vi "0506_Identificador_QR.vi"() -> (27 "error out":errorcluster)   [LabVIEW 2017]
uses:
  <vilib>/userdefined/High Color/IMAQdx.ctl
  <vilib>/vision/Instrument.llb/QR Code Search Options.ctl
  <vilib>/vision/Instrument.llb/Demodulation Mode.ctl
  <vilib>/vision/Instrument.llb/Cell Sample Size.ctl
  <vilib>/vision/Instrument.llb/Cell Filter Mode.ctl
  <vilib>/vision/Instrument.llb/QR Code Description Options.ctl
  <vilib>/vision/Instrument.llb/Data Matrix Polarity.ctl
  <vilib>/vision/Instrument.llb/QR Code Model Type.ctl
  <vilib>/vision/driver/IMAQdx.llb/IMAQdx Acquisition Mode.ctl
  <vilib>/vision/driver/IMAQdx.llb/IMAQdx Buffer Number Mode.ctl
  <vilib>/vision/NI_Vision_Development_Module.lvlib
  <vilib>/vision/driver/NI_Vision_Acquisition_Software.lvlib
panel:
  out "Table Control":string[][](table)
  in  "Boolean":bool
  out "dt":dbl
  in  "QR Description Options":T1={"Matrix Size (cells)"=0, "Barcode Polarity"=-2, "Mirror Mode"=0, "QR Model"=3} {"Mirror Mode" items=["Auto-detect"=-2, "Normal"=0, "Mirrored"=1]; "Matrix Size (cells)" items=["Auto-detect"=0, "11x11 - Version 1 (Micro QR Only)"=11, "13x13 - Version 2 (Micro QR Only)"=13, "15x15 - Version 3 (Micro QR Only)"=15, "17x17 - Version 4 (Micro QR Only)"=17, "21x21 - Version 1"=21, "25x25 - Version 2"=25, "29x29 - Version 3"=29, "33x33 - Version 4"=33, "37x37 - Version 5"=37, "41x41 - Version 6"=41, "45x45 - Version 7"=45, "49x49 - Version 8"=49, "53x53 - Version 9"=53, "57x57 - Version 10"=57, "61x61 - Version 11"=61, "65x65 - Version 12"=65, "69x69 - Version 13"=69, "73x73 - Version 14"=73, "77x77 - Version 15"=77, "81x81 - Version 16"=81, "85x85 - Version 17"=85, "89x89 - Version 18"=89, "93x93 - Version 19"=93, "97x97 - Version 20"=97, "101x101 - Version 21"=101, "105x105 - Version 22"=105, "109x109 - Version 23"=109, "113x113 - Version 24"=113, "117x117 - Version 25"=117, "121x121 - Version 26"=121, "125x125 - Version 27"=125, "129x129 - Version 28"=129, "133x133 - Version 29"=133, "137x137 - Version 30"=137, "141x141 - Version 31"=141, "145x145 - Version 32"=145, "149x149 - Version 33"=149, "153x153 - Version 34"=153, "157x157 - Version 35"=157, "161x161 - Version 36"=161, "165x165 - Version 37"=165, "169x169 -  Version 38"=169, "173x173 - Version 39"=173, "177x177 - Version 40"=177]; "QR Model" items=["Auto-detect", "Micro", "Model 1", "Model 2"]; "Barcode Polarity" items=["Auto-detect"=-2, "Black on White"=0, "White on Black"=1]}
  in  "QR Search Options":T4={"Rotation Mode"=enum."Unlimited", "Skip Location?"=FALSE, "Edge Threshold"=30, "Demodulation Mode"=0, "Cell Sample Size"=-2, "Cell Filter Mode"=0, "Skew Degrees Allowed"=5} {"Cell Filter Mode" items=["Auto-detect"=-2, "Average"=0, "Median"=1, "Central Average"=2, "High Average"=3, "Low Average"=4, "Very High Average"=5, "Very Low Average"=6, "All Filters"=8]; "Cell Sample Size" items=["Auto-detect"=-2, "1x1"=1, "2x2"=2, "3x3"=3, "4x4"=4, "5x5"=5, "6x6"=6, "7x7"=7]; "Demodulation Mode" items=["Auto-detect"=-2, "Histogram"=0, "Local Contrast"=1, "Combination"=2, "All"=3]}
  in  "Threshold":cluster{"Lower value":sgl, "Upper value":sgl}={"Lower value"=0.0, "Upper value"=201.0219} {"Upper value" scale=0.0..255.0; "Lower value" scale=0.0..255.0}
  out "Image Out 2":T8(plugin-control)
  in  "Câmera":T9="cam1"
  in  "Stop Button":bool
  out "Image Out":T8(plugin-control)
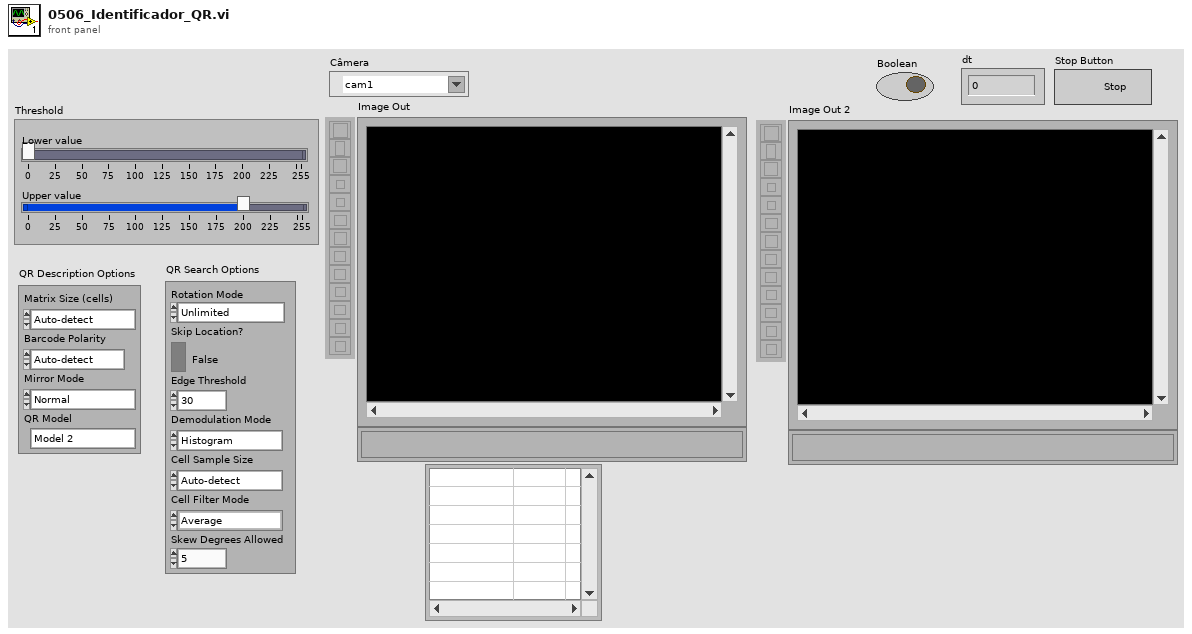
[diagram p1: front panel]
types:
  T1 = typedef "QR Code Description Options.ctl" = cluster{"Matrix Size (cells)":i32, "Barcode Polarity":T2, "Mirror Mode":i32, "QR Model":T3}
  T2 = typedef "Data Matrix Polarity.ctl" = i32
  T3 = typedef "QR Code Model Type.ctl" = i32
  T4 = typedef "QR Code Search Options.ctl" = cluster{"Rotation Mode":enum32{"Unlimited", "0 Degrees", "90 Degrees", "180 Degrees", "270 Degrees"}, "Skip Location?":bool, "Edge Threshold":u32, "Demodulation Mode":T5, "Cell Sample Size":T6, "Cell Filter Mode":T7, "Skew Degrees Allowed":u32}
  T5 = typedef "Demodulation Mode.ctl" = i32
  T6 = typedef "Cell Sample Size.ctl" = i32
  T7 = typedef "Cell Filter Mode.ctl" = i32
  T8 = typedef "IMAQ Image.ctl" = refnum<image>
  T9 = typedef "IMAQdx.ctl" = refnum<k21>
  T10 = typedef "Image Type" = u32
  T11 = typedef "NI_Vision_Acquisition_Software.lvlib/IMAQdx Acquisition Mode.ctl" = enum32{"One Shot", "Continuous"}
  T12 = typedef "NI_Vision_Acquisition_Software.lvlib/IMAQdx Buffer Number Mode.ctl" = enum32{"Next", "Last", "Buffer Number", "Every", "Last New"}
  T13 = cluster{"Global Rectangle":i32[], "Contours":cluster{"Contour Type":u32, "ROI Type":u32, "Points":i32[]}[]}
  T14 = typedef "QR Code Report.ctl" = cluster{"Found?":bool, "Data":string, "Bounding Box":cluster{"x":sgl, "y":sgl}[], "Errors Corrected":u32, "Dimensions (Rows/Cols)":u32, "Version":u32, "QR Model":T3, "Stream Mode":T15, "Barcode Polarity":T2, "Mirrored?":bool, "Append Stream Position":u32, "Size of Append Stream":u32, "First EAN-128 ID":i32, "First Alternate Language ID":i32, "Append Stream ID":u32, "Minimum Edge Strength":u32, "Demodulation Mode":T5, "Cell Sample Size":T6, "Cell Filter Mode":T7}
  T15 = typedef "QR Code Stream Mode Type.ctl" = i32
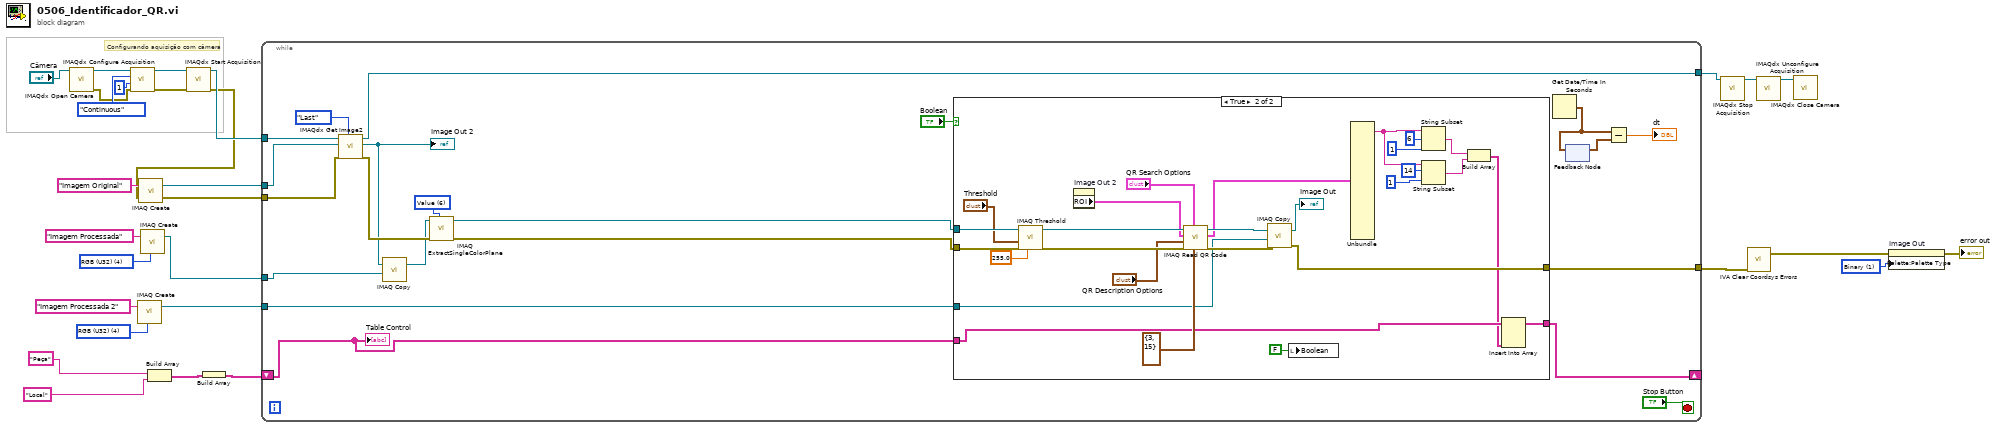
[diagram p0: block diagram]
diagram:
  w7 = T10 4 items=["Grayscale (U8)", "Grayscale (I16)", "Grayscale (SGL)", "Complex (CSG)", "RGB (U32)", "HSL (U32)", "RGB (U64)", "Grayscale (U16)"] ("Image Type")
  w14 = u32 1 items=["Grayscale", "Binary", "Gradient", "Rainbow", "Temperature", "User Defined", "Binary 16 Bit", "Gradient 16 Bit", "Rainbow 16 Bit", "Temperature 16 Bit", "User Defined 16 Bit"] ("Palette Type")
  w23 = T10 4 items=["Grayscale (U8)", "Grayscale (I16)", "Grayscale (SGL)", "Complex (CSG)", "RGB (U32)", "HSL (U32)", "RGB (U64)", "Grayscale (U16)"] ("Image Type")
  # "Configurando aquisição com câmera"
  n1 = call <vilib>:"IMAQdx Open Camera.vi"("Session In"="Câmera") -> ("error out"=w19:errorcluster, "Session Out"=w29:T9)  [unwired: 9 in]
  n2 = call <vilib>:"IMAQdx Configure Acquisition.vi"("error in"=w19, "Number of Buffers"=u32 1, "Continuous?"=IMAQdx_Acquisition_Mode."Continuous", "Session In"=w29) -> ("error out"=w20:errorcluster, "Session Out"=w28:T9)  [unwired: 6 in]
  n3 = call "IMAQ Create"("Image Name"="Imagem Processada 2", "Image Type"=w7) -> ("New Image"=w5:T8)  [unwired: 3 in, 1 out]
  n4 = call "IMAQ Create"("Image Name"="Imagem Processada", "Image Type"=w23) -> ("New Image"=w8:T8)  [unwired: 3 in, 1 out]
  n5 = Build Array("Peça" ("string"), "Local" ("string")) -> (w2:string[])
  n6 = call <vilib>:"IMAQdx Start Acquisition.vi"("error in"=w20, "Session In"=w28) -> ("error out"=w18:errorcluster, "Session Out"=w21:T9)  [unwired: 8 in]
  n7 = call "IMAQ Create"("Image Name"="Imagem Original", "error in (no error)"=w18) -> ("New Image"=w22:T8, "error out"=w17:errorcluster)  [unwired: 3 in]
  n8 = Build Array(w2) -> (w1:string[][])
  n9 = while {
    tunnel: w22 -> [w46]
    tunnel: w21 -> [w45]
    tunnel: w17 -> [w44]
    tunnel: [w41] -> w13
    tunnel: [w40] -> w10
    tunnel: w8 -> [w39]
    tunnel: w5 -> [w32]
    shift-right: [w30] -> _
    shift-left: w1 -> [w31]
    stop <- "Stop Button" stop-if-true
    w50 = 6 items=["Red", "Green", "Blue", "Hue", "Saturation", "Luminance", "Value", "Intensity"] ("Color Plane")
    n10 = call <vilib>:"IMAQdx Get Image2.vi"("Buffer Number Mode (Next)"=IMAQdx_Buffer_Number_Mode."Last", "error in"=w44, "Image In"=w46, "Session In"=w45) -> ("error out"=w43:errorcluster, "Image Out"=w37:T8, "Session Out"=w40:T9)  [unwired: 4 in, 1 out]
    "Image Out 2" <- w37
    n11 = call "IMAQ Copy"("Image Dst"=w39, "Image Src"=w37) -> ("Image Dst Out"=w38:T8)  [unwired: 4 in, 1 out]
    n12 = call "IMAQ ExtractSingleColorPlane"("Color Plane"=w50, "error in (no error)"=w43, "Image Src"=w38) -> ("error out"=w49:errorcluster, "Image Dst Out"=w48:T8)  [unwired: 1 in, 6 out]
    n13 = case shown="True" "Boolean" {
      tunnel: w49 -> [w52 w79]
      tunnel: w48 -> [_ w78]
      tunnel: [w52 w65] -> w41
      tunnel: w32 -> [_ w64]
      tunnel: w31 -> [w51 w55]
      tunnel: [w51 w54] -> w30
      frame False {
      }
      frame True {
        n14 = call "IMAQ Threshold"("Replace Value"=sgl 255.0, "error in (no error)"=w79, "Range"="Threshold", "Image Src"=w78) -> ("error out"=w74:errorcluster, "Image Dst Out"=w75:T8)  [unwired: 2 in, 4 out]
        n15 = property on="Image Out 2" class="ImageControl"() -> ("ROI"=w70:T13)  [unwired: 2 in, 2 out]
        n16 = call "IMAQ Read QR Code"("QR Code Cell Size (pixels)"=cluster{"Minimum Size":u32, "Maximum Size":u32} {"Minimum Size"=3, "Maximum Size"=15}, "QR Search Options"="QR Search Options", "error in (no error)"=w74, "QR Description Options"="QR Description Options", "ROI Descriptor"=w70, "Image"=w75) -> ("error out"=w66:errorcluster, "QR Code Report"=w63:T14, "Image (duplicate)"=w67:T8)  [unwired: 1 in, 2 out]
        n17 = call "IMAQ Copy"("error in (no error)"=w66, "Image Dst"=w64, "Image Src"=w67) -> ("error out"=w65:errorcluster, "Image Dst Out"=→"Image Out":T8)  [unwired: 3 in]
        n18 = local write "Boolean"(FALSE ("Boolean")) -> ()
        n19 = Unbundle(w63) -> ("Data"=w60:string)  [unwired: 18 out]
        n20 = String Subset(string=w60, offset (0)=6, length (rest)=1 ("length (rest)")) -> (substring=w57:string)
        n21 = String Subset(string=w60, offset (0)=14, length (rest)=1 ("length (rest)")) -> (substring=w56:string)
        n22 = Build Array(w57, w56) -> (w53:string[])
        n23 = Insert Into Array(array=w55, new element=w53) -> (w54:string[][])  [unwired: 2 in]
      }
    }
    n24 = Get Date/Time In Seconds() -> (seconds since 1Jan1904=w35:timestamp)
    n25 = feedback #1() -> (w36:timestamp)  [unwired: 1 in]
    n26 = feedback-in #1(w35) -> ()
    n27 = Subtract(x=w35, y=w36) -> (x-y=→"dt":dbl)
    "Table Control" <- w31
  }
  n28 = call <vilib>:"IMAQdx Stop Acquisition.vi"("Session In"=w10) -> ("Session Out"=w12:T9)  [unwired: 9 in, 1 out]
  n29 = call <vilib>:"IVA Clear Coordsys Errors.vi"("error in (no error)"=w13) -> ("error out"=w15:errorcluster)  [unwired: 10 in]
  n30 = call <vilib>:"IMAQdx Unconfigure Acquisition.vi"("Session In"=w12) -> ("Session Out"=w11:T9)  [unwired: 9 in, 1 out]
  n31 = call <vilib>:"IMAQdx Close Camera.vi"("Session In"=w11) -> ()  [unwired: 10 in, 1 out]
  n32 = property on="Image Out" class="ImageControl"(error in=w15, "Palette:Palette Type"=w14) -> (error out=→"error out":errorcluster)  [unwired: 1 in, 1 out]
